vi "Periodic Tasks.vi"(8 "error in":errorcluster) -> ()   [LabVIEW 2012]
doc: "This VI runs in parallel to other tasks. It can contain as many user-defined periodic loops as you need. These can carry out PID or other sorts of timed response."
uses:
  <vilib>/Rock Robotics/SystemInterfaces/Utilities/FPGA_UtilitiesLED Source.ctl
  <vilib>/Rock Robotics/SystemInterfaces/Utilities/FPGA_UtilitiesLED State.ctl
  <vilib>/Rock Robotics/WPI/Relay/WPI_RelayValue.ctl
  <vilib>/Rock Robotics/WPI/RobotDrive/WPI_RobotDriveGetSetRefNum.vi
  Robot Global Data.vi
  <vilib>/Rock Robotics/WPI/Joystick/WPI_JoystickGetSetRefNum.vi
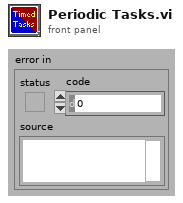
[diagram p1: front panel]
types:
  T1 = typedef "WPI_JoystickDevRef.ctl" = cluster{"Device":T2}
  T2 = typedef "WPI_JoystickDeviceEnum.ctl" = enum16{"USB 1", "USB 2", "USB 3", "USB 4", "Kinect 1", "Kinect 2"}
  T3 = typedef "WPI_RobotDriveDevRef.ctl" = cluster{"DevStatus":errorcluster, "Motors[]":T4[], "Square Inputs":bool, "Max Output":dbl, "Isochronous":bool}
  T4 = typedef "WPI_MotorControlDeviceRef.ctl" = cluster{"DeviceStatus":errorcluster, "Type":enum16{"PWM", "CAN"}, "PWM":cluster{"Digital Module":T5, "PWM Channel":T6, "DeadBand":T7}, "CAN":cluster{"Device Number":u8, "Control Mode":T8, "Semaphore":T9, "Max Vout":dbl}, "Invert":bool, "TransformRef":T10, "InvTransformRef":T10}
  T5 = typedef "FPGA_TypedefDigitalModule.ctl" = enum16{"Digital Module 1", "Digital Module 2"}
  T6 = typedef "FPGA_DIOPWMChannel.ctl" = enum8{"PWM 1", "PWM 2", "PWM 3", "PWM 4", "PWM 5", "PWM 6", "PWM 7", "PWM 8", "PWM 9", "PWM 10", "Invalid"}
  T7 = typedef "WPI_PWMDeadband.ctl" = cluster{"Name":string, "maxPositivePwm":i32, "minPositivePwm":i32, "centerPwm":i32, "maxNegativePwm":i32, "minNegativePwm":i32, "angularRange":u16}
  T8 = typedef "WPI_CANJaguar_ControlMode.ctl" = enum8{"Percent VBus", "Current", "Speed", "Position", "Voltage"}
  T9 = typedef "Semaphore RefNum" = refnum<k1>
  T10 = typedef "WPI_PWMTransform_ConPane.ctl" = refnum<vi>
  T11 = cluster{"JoystickDevRef":T1, "RobotDriveDevRef":T3}
  T12 = typedef "WPI_RelayValue.ctl" = enum16{"Off", "On", "Forward", "Reverse"}
  T13 = typedef "WPI_RelayDevRef.ctl" = cluster{"DevStatus":errorcluster, "Relay Channel":T14, "Digital Module":T5, "Relay Direction":T15}
  T14 = typedef "FPGA_DIORelayChannel.ctl" = enum8{"Relay 1", "Relay 2", "Relay 3", "Relay 4", "Relay 5", "Relay 6", "Relay 7", "Relay 8", "Invalid"}
  T15 = typedef "WPI_RelayDirection.ctl" = enum16{"Both directions", "Forward only", "Reverse only"}
  T16 = typedef "FPGA_UtilitiesLED State.ctl" = enum16{"Off", "On", "Toggle"}
  T17 = typedef "FPGA_UtilitiesLED Source.ctl" = enum16{"User LED", "FPGA LED"}
  T18 = typedef "WPI_CompressorDevRef.ctl" = cluster{"DevStatus":errorcluster, "DigitalInputDevRef":T19, "RelayDevRef":T13}
  T19 = typedef "WPI_DigitalInputDevRef.ctl" = cluster{"DevStatus":errorcluster, "DIO Channel":T20, "Digital Module":T5}
  T20 = typedef "FPGA_DIOChannel.ctl" = enum8{"DIO 1", "DIO 2", "DIO 3", "DIO 4", "DIO 5", "DIO 6", "DIO 7", "DIO 8", "DIO 9", "DIO 10", "DIO 11", "DIO 12", "DIO 13", "DIO 14", "Invalid"}
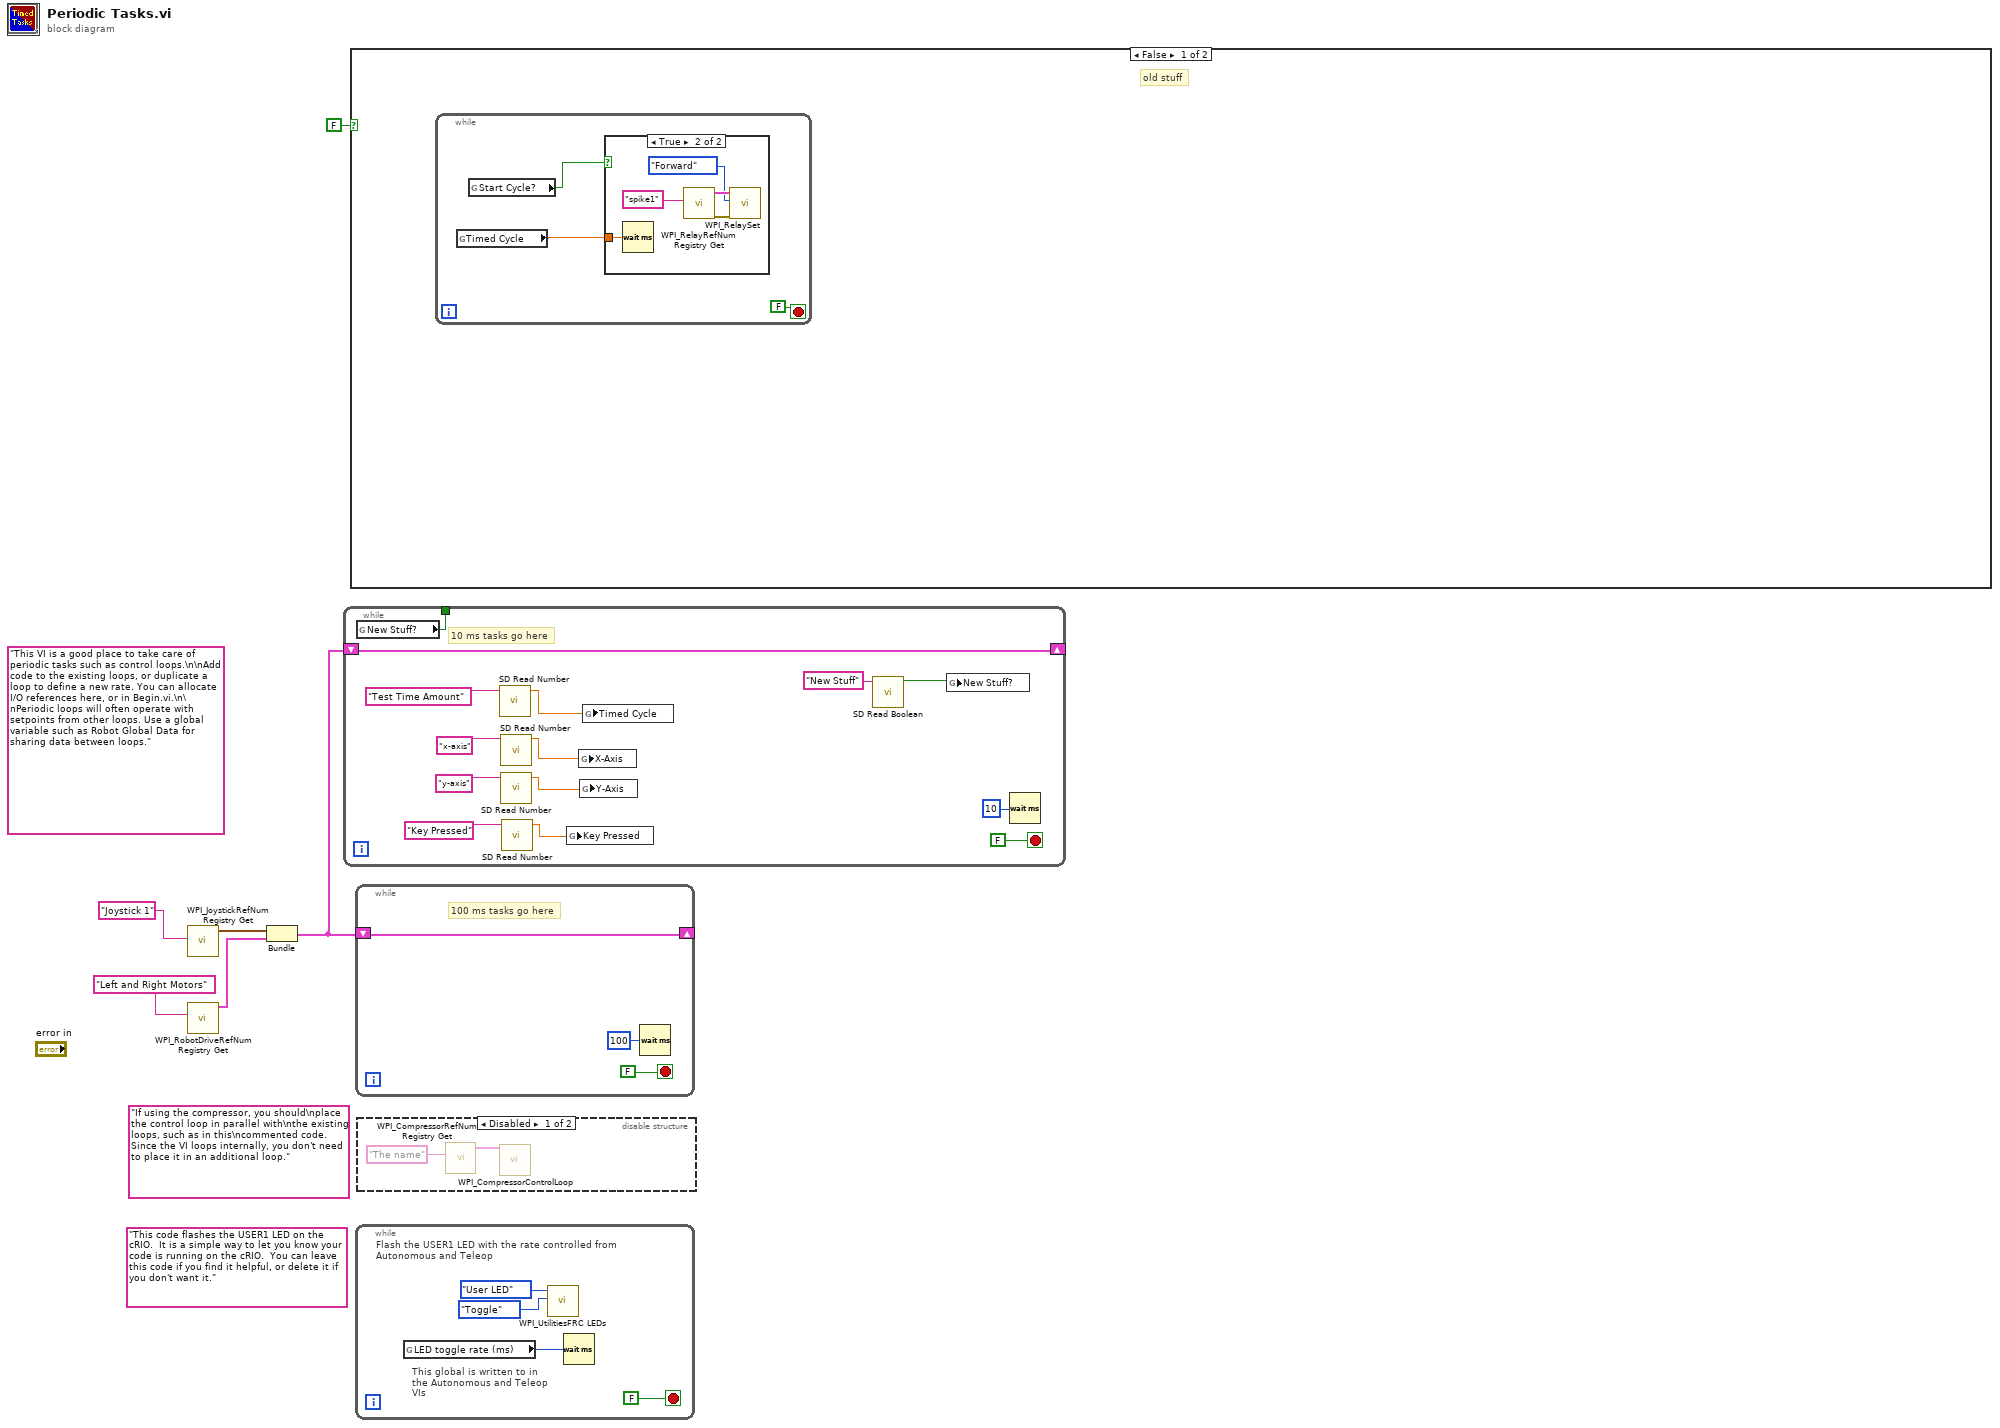
[diagram p0: block diagram]
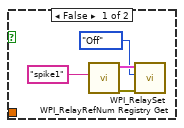
[diagram p2: hidden frame]
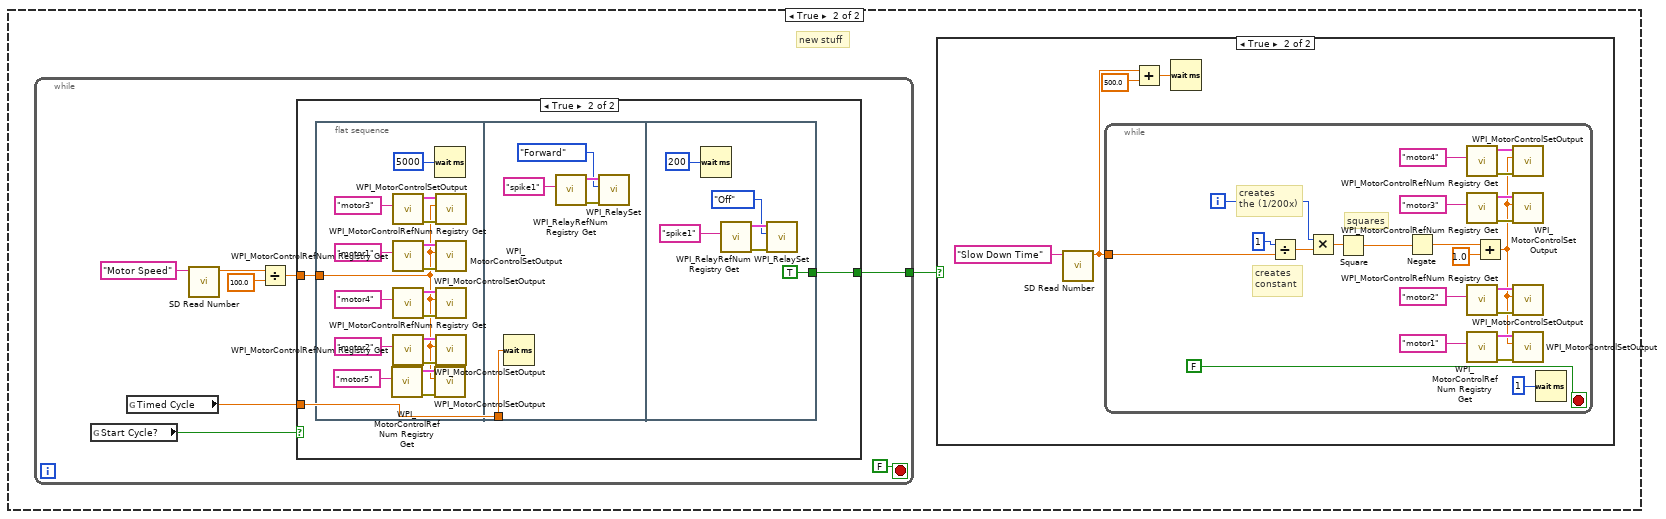
[diagram p3: hidden frame]
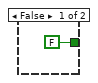
[diagram p5: hidden frame]
diagram:
  (unwired) "If using the compressor, you should\nplace the control loop in parallel with\nthe existing loops, such as in this\ncommented code. Since the VI loops internally, you don't need to place it in an additional loop."
  (unwired) "This code flashes the USER1 LED on the cRIO.  It is a simple way to let you know your code is running on the cRIO.  You can leave this code if you find it helpful, or delete it if you don't want it."
  (unwired) "This VI is a good place to take care of periodic tasks such as control loops.\n\nAdd code to the existing loops, or duplicate a loop to define a new rate. You can allocate I/O references here, or in Begin.vi.\n\nPeriodic loops will often operate with setpoints from other loops. Use a global variable such as Robot Global Data for sharing data between loops."
  n1 = call <vilib>:"WPI_JoystickRefNum Registry Get.vi"("refnum name"="Joystick 1") -> ("JoystickDevRef"=w4:T1)  [unwired: 1 in, 9 out]
  n2 = call <vilib>:"WPI_RobotDriveRefNum Registry Get.vi"("refnum name"="Left and Right Motors") -> ("RobotDriveDevRef"=w3:T3)  [unwired: 1 in, 9 out]
  n3 = Bundle("JoystickDevRef"=w4, "RobotDriveDevRef"=w3) -> (w2:T11)  [unwired: 1 out]
  n4 = while {
    shift-right: [w18] -> _
    shift-left: w2 -> [w18]
    tunnel: [w7] -> _
    stop <- FALSE stop-if-true
    # "10 ms tasks go here"
    n5 = global read "Robot Global Data.vi" "New Stuff?"() -> (w7:bool)
    n6 = call <vilib>:"SD Read Number.vi"("Name"="Test Time Amount" ("refnum name")) -> ("Numeric"=w16:dbl)  [unwired: 8 in, 2 out]
    n7 = call <vilib>:"SD Read Number.vi"("Name"="x-axis" ("refnum name")) -> ("Numeric"=w13:dbl)  [unwired: 8 in, 2 out]
    n8 = call <vilib>:"SD Read Number.vi"("Name"="y-axis" ("refnum name")) -> ("Numeric"=w12:dbl)  [unwired: 8 in, 2 out]
    n9 = call <vilib>:"SD Read Number.vi"("Name"="Key Pressed" ("refnum name")) -> ("Numeric"=w10:dbl)  [unwired: 8 in, 2 out]
    n10 = global write "Robot Global Data.vi" "Key Pressed"(w10) -> ()
    n11 = global write "Robot Global Data.vi" "X-Axis"(w13) -> ()
    n12 = global write "Robot Global Data.vi" "Y-Axis"(w12) -> ()
    n13 = global write "Robot Global Data.vi" "Timed Cycle"(w16) -> ()
    n14 = call <vilib>:"SD Read Boolean.vi"("Name"="New Stuff") -> ("Boolean"=w8:bool)  [unwired: 8 in, 2 out]
    n15 = global write "Robot Global Data.vi" "New Stuff?"(w8) -> ()
    n16 = Wait (ms)(milliseconds to wait=u32 10) -> ()  [unwired: 1 out]
  }
  n17 = case shown="False" FALSE {
    frame False {
      # "old stuff"
      n18 = while {
        stop <- FALSE stop-if-true
        n19 = global read "Robot Global Data.vi" "Timed Cycle"() -> (w22:dbl)
        n20 = global read "Robot Global Data.vi" "Start Cycle?"() -> (w21:bool)
        n21 = case shown="True" w21 {
          tunnel: w22 -> [_ w32]
          frame False {
            n22 = call <vilib>:"WPI_RelayRefNum Registry Get.vi"("refnum name"="spike1") -> ("error out"=w27:errorcluster, "RelayDevRef"=w26:T13)  [unwired: 9 in]
            n23 = call <vilib>:"WPI_RelaySet.vi"("error in (no error)"=w27, "RelayValue"=WPI_RelayValue."Off", "RelayDevRef"=w26) -> ()  [unwired: 7 in, 2 out]
          }
          frame True {
            n24 = Wait (ms)(milliseconds to wait=w32) -> ()  [unwired: 1 out]
            n25 = call <vilib>:"WPI_RelayRefNum Registry Get.vi"("refnum name"="spike1") -> ("error out"=w31:errorcluster, "RelayDevRef"=w30:T13)  [unwired: 9 in]
            n26 = call <vilib>:"WPI_RelaySet.vi"("error in (no error)"=w31, "RelayValue"=WPI_RelayValue."Forward", "RelayDevRef"=w30) -> ()  [unwired: 7 in, 2 out]
          }
        }
      }
    }
    frame True {
      # "new stuff"
      n27 = while {
        tunnel: [w61] -> w33
        stop <- FALSE stop-if-true
        n28 = global read "Robot Global Data.vi" "Start Cycle?"() -> (w67:bool)
        n29 = global read "Robot Global Data.vi" "Timed Cycle"() -> (w66:dbl)
        n30 = call <vilib>:"SD Read Number.vi"("Name"="Motor Speed" ("refnum name")) -> ("Numeric"=w64:dbl)  [unwired: 8 in, 2 out]
        n31 = Divide(x=w64, y=100.0) -> (x/y=w62:dbl)
        n32 = case shown="True" w67 {
          tunnel: w66 -> [_ w71]
          tunnel: w62 -> [_ w72]
          tunnel: [FALSE w70] -> w61
          frame False {
          }
          frame True {
            n33 = flat-sequence {
              tunnel: w72 -> [w73]
              tunnel: w71 -> [w90]
              tunnel: [TRUE] -> w70
              frame #0 {
                n34 = call <vilib>:"WPI_MotorControlRefNum Registry Get.vi"("refnum name"="motor5") -> ("error out"=w75:errorcluster, "MotorControlDevRef"=w76:T4)  [unwired: 9 in]
                n35 = call <vilib>:"WPI_MotorControlRefNum Registry Get.vi"("refnum name"="motor3") -> ("error out"=w83:errorcluster, "MotorControlDevRef"=w77:T4)  [unwired: 9 in]
                n36 = call <vilib>:"WPI_MotorControlRefNum Registry Get.vi"("refnum name"="motor1") -> ("error out"=w88:errorcluster, "MotorControlDevRef"=w89:T4)  [unwired: 9 in]
                n37 = call <vilib>:"WPI_MotorControlRefNum Registry Get.vi"("refnum name"="motor4") -> ("error out"=w80:errorcluster, "MotorControlDevRef"=w81:T4)  [unwired: 9 in]
                n38 = call <vilib>:"WPI_MotorControlRefNum Registry Get.vi"("refnum name"="motor2") -> ("error out"=w85:errorcluster, "MotorControlDevRef"=w86:T4)  [unwired: 9 in]
                n39 = Wait (ms)(milliseconds to wait=u32 5000) -> ()  [unwired: 1 out]
                n40 = call <vilib>:"WPI_MotorControlSetOutput.vi"("error in (no error)"=w75, "Output"=w73, "MotorControlDevRef"=w76) -> ()  [unwired: 6 in, 3 out]
                n41 = call <vilib>:"WPI_MotorControlSetOutput.vi"("error in (no error)"=w83, "Output"=w73, "MotorControlDevRef"=w77) -> ()  [unwired: 6 in, 3 out]
                n42 = call <vilib>:"WPI_MotorControlSetOutput.vi"("error in (no error)"=w88, "Output"=w73, "MotorControlDevRef"=w89) -> ()  [unwired: 6 in, 3 out]
                n43 = call <vilib>:"WPI_MotorControlSetOutput.vi"("error in (no error)"=w80, "Output"=w73, "MotorControlDevRef"=w81) -> ()  [unwired: 6 in, 3 out]
                n44 = call <vilib>:"WPI_MotorControlSetOutput.vi"("error in (no error)"=w85, "Output"=w73, "MotorControlDevRef"=w86) -> ()  [unwired: 6 in, 3 out]
              }
              frame #1 {
                n45 = Wait (ms)(milliseconds to wait=w90) -> ()  [unwired: 1 out]
                n46 = call <vilib>:"WPI_RelayRefNum Registry Get.vi"("refnum name"="spike1") -> ("error out"=w94:errorcluster, "RelayDevRef"=w93:T13)  [unwired: 9 in]
                n47 = call <vilib>:"WPI_RelaySet.vi"("error in (no error)"=w94, "RelayValue"=WPI_RelayValue."Forward", "RelayDevRef"=w93) -> ()  [unwired: 7 in, 2 out]
              }
              frame #2 {
                n48 = Wait (ms)(milliseconds to wait=u32 200) -> ()  [unwired: 1 out]
                n49 = call <vilib>:"WPI_RelayRefNum Registry Get.vi"("refnum name"="spike1") -> ("error out"=w100:errorcluster, "RelayDevRef"=w99:T13)  [unwired: 9 in]
                n50 = call <vilib>:"WPI_RelaySet.vi"("error in (no error)"=w100, "RelayValue"=WPI_RelayValue."Off", "RelayDevRef"=w99) -> ()  [unwired: 7 in, 2 out]
              }
            }
          }
        }
      }
      n51 = case shown="True" w33 {
        frame False {
        }
        frame True {
          n52 = call <vilib>:"SD Read Number.vi"("Name"="Slow Down Time" ("refnum name")) -> ("Numeric"=w36:dbl)  [unwired: 8 in, 2 out]
          n53 = while {
            tunnel: w36 -> [w40]
            i -> [w39]
            stop <- FALSE stop-if-true
            # "squares"
            # "creates \nthe (1/200x)"
            # "creates\nconstant"
            n54 = Divide(x=u32 1 ("milliseconds to wait"), y=w40) -> (x/y=w46:dbl)
            n55 = Multiply(x=w39, y=w46) -> (x*y=w47:dbl)
            n56 = Square(x=w47) -> (x^2=w44:dbl)
            n57 = Negate(x=w44) -> (-x=w43:dbl)
            n58 = call <vilib>:"WPI_MotorControlRefNum Registry Get.vi"("refnum name"="motor4") -> ("error out"=w49:errorcluster, "MotorControlDevRef"=w50:T4)  [unwired: 9 in]
            n59 = call <vilib>:"WPI_MotorControlRefNum Registry Get.vi"("refnum name"="motor3") -> ("error out"=w52:errorcluster, "MotorControlDevRef"=w53:T4)  [unwired: 9 in]
            n60 = call <vilib>:"WPI_MotorControlRefNum Registry Get.vi"("refnum name"="motor2") -> ("error out"=w55:errorcluster, "MotorControlDevRef"=w56:T4)  [unwired: 9 in]
            n61 = call <vilib>:"WPI_MotorControlRefNum Registry Get.vi"("refnum name"="motor1") -> ("error out"=w58:errorcluster, "MotorControlDevRef"=w59:T4)  [unwired: 9 in]
            n62 = Add(x=w43, y=1.0) -> (x+y=w41:dbl)
            n63 = call <vilib>:"WPI_MotorControlSetOutput.vi"("error in (no error)"=w49, "Output"=w41, "MotorControlDevRef"=w50) -> ()  [unwired: 6 in, 3 out]
            n64 = call <vilib>:"WPI_MotorControlSetOutput.vi"("error in (no error)"=w52, "Output"=w41, "MotorControlDevRef"=w53) -> ()  [unwired: 6 in, 3 out]
            n65 = call <vilib>:"WPI_MotorControlSetOutput.vi"("error in (no error)"=w55, "Output"=w41, "MotorControlDevRef"=w56) -> ()  [unwired: 6 in, 3 out]
            n66 = call <vilib>:"WPI_MotorControlSetOutput.vi"("error in (no error)"=w58, "Output"=w41, "MotorControlDevRef"=w59) -> ()  [unwired: 6 in, 3 out]
            n67 = Wait (ms)(milliseconds to wait=u32 1) -> ()  [unwired: 1 out]
          }
          n68 = Add(x=w36, y=500.0) -> (x+y=w34:dbl)
          n69 = Wait (ms)(milliseconds to wait=w34) -> ()  [unwired: 1 out]
        }
      }
    }
  }
  n70 = while {
    shift-right: [w101] -> _
    shift-left: w2 -> [w101]
    stop <- FALSE stop-if-true
    # "100 ms tasks go here"
    n71 = Wait (ms)(milliseconds to wait=u32 100) -> ()  [unwired: 1 out]
  }
  n72 = while {
    stop <- FALSE stop-if-true
    # "This global is written to in the Autonomous and Teleop VIs"
    # "Flash the USER1 LED with the rate controlled from Autonomous and Teleop"
    n73 = global read "Robot Global Data.vi" "LED toggle rate (ms)"() -> (w104:u32)
    n74 = call <vilib>:"WPI_UtilitiesFRC LEDs.vi"("State"=FPGA_UtilitiesLED_State."Toggle", "LED Type"=FPGA_UtilitiesLED_Source."User LED") -> ()  [unwired: 1 in, 9 out]
    n75 = Wait (ms)(milliseconds to wait=w104) -> ()  [unwired: 1 out]
  }
  n76 = disable-structure shown="Disabled" {
    frame Disabled {
      n77 = call <vilib>:"WPI_CompressorRefNum Registry Get.vi"("refnum name"="The name") -> ("CompressorDevRef"=w109:T18)  [unwired: 9 in, 1 out]
      n78 = call <vilib>:"WPI_CompressorControlLoop.vi"("CompressorDevRef"=w109) -> ()  [unwired: 11 in]
    }
    frame Enabled {
    }
  }
